vi "Workspace.Initialize.vi"(9 "State Variables in":T1, 10 "Item.Data":T8, 11 "NIVS.Gateway IP Address":string) -> (0 "error out":errorcluster, 3 "State Variables out":T1)   [LabVIEW 2019, in "Protection and Counter Workspace Shared.lvlib"]
uses:
  Protection and Counter Workspace Shared.lvlib
  <vilib>/NI VeriStand/Display Template Support/DisplayTemplateSupport.llb/cluster_Screen Item Settings.ctl
  <vilib>/NI VeriStand/Display Template Support/DisplayTemplateSupport.llb/cluster_Graph Scale Settings.ctl
  <vilib>/NI VeriStand/Display Template Support/DisplayTemplateSupport.llb/cluster_Graph Plot Settings.ctl
  Types/Workspace.State.ctl
  Types/UI.Refs.ctl
  SubModules/CAN-Streaming-Support/Source/Addon/Addon Shared/Types/Type Filter.ctl
  <vilib>/NI VeriStand/Display Template Support/DisplayTemplateSupport.llb/enum_Display Template Handler Minimal To Workspace.ctl
  Types/Workspace.SavedState.ctl
  NationalInstruments.VeriStand.SystemStorage
  <vilib>/NI VeriStand/Execution/Workspace/WorkspaceAPI.ctl
  NationalInstruments.VeriStand.ClientAPI
  <vilib>/NI VeriStand/Display Template Support/DisplayTemplateSupport.llb/enum_Display Template Handler Minimal To Widget Msg.ctl
  <vilib>/NI VeriStand/Execution/Workspace/SystemStateRegEventRef.ctl
  <vilib>/NI VeriStand/Execution/Workspace/Target State Info.ctl
  <vilib>/NI VeriStand/Execution/Workspace/Target State.ctl
  <vilib>/NI VeriStand/Execution/Workspace/SystemStateEventRef.ctl
  SubModules/CAN-Streaming-Support/Source/UIs/Workspace Shared/Types/Host Stream Queue Refs.ctl
  SubModules/CAN-Streaming-Support/Source/UIs/Workspace Shared/Types/Host Stream Queue Type.ctl
  SubModules/CAN-Streaming-Support/Source/UIs/Workspace Shared/Types/Host Stream Queue Command.ctl
  <vilib>/xnet/xnet.llb/XNET Frame CAN.ctl
  <vilib>/xnet/xnet.llb/XNET Frame Type CAN.ctl
  <vilib>/NI VeriStand/Execution/Workspace/NI_VS Workspace ExecutionAPI.lvlib
  SubModules/CAN-Streaming-Support/Source/UIs/Workspace Shared/CAN Stream Support Workspace Shared.lvlib
  SubModules/CAN-Streaming-Support/Source/Addon/Addon Shared/CAN Stream Support Shared.lvlib
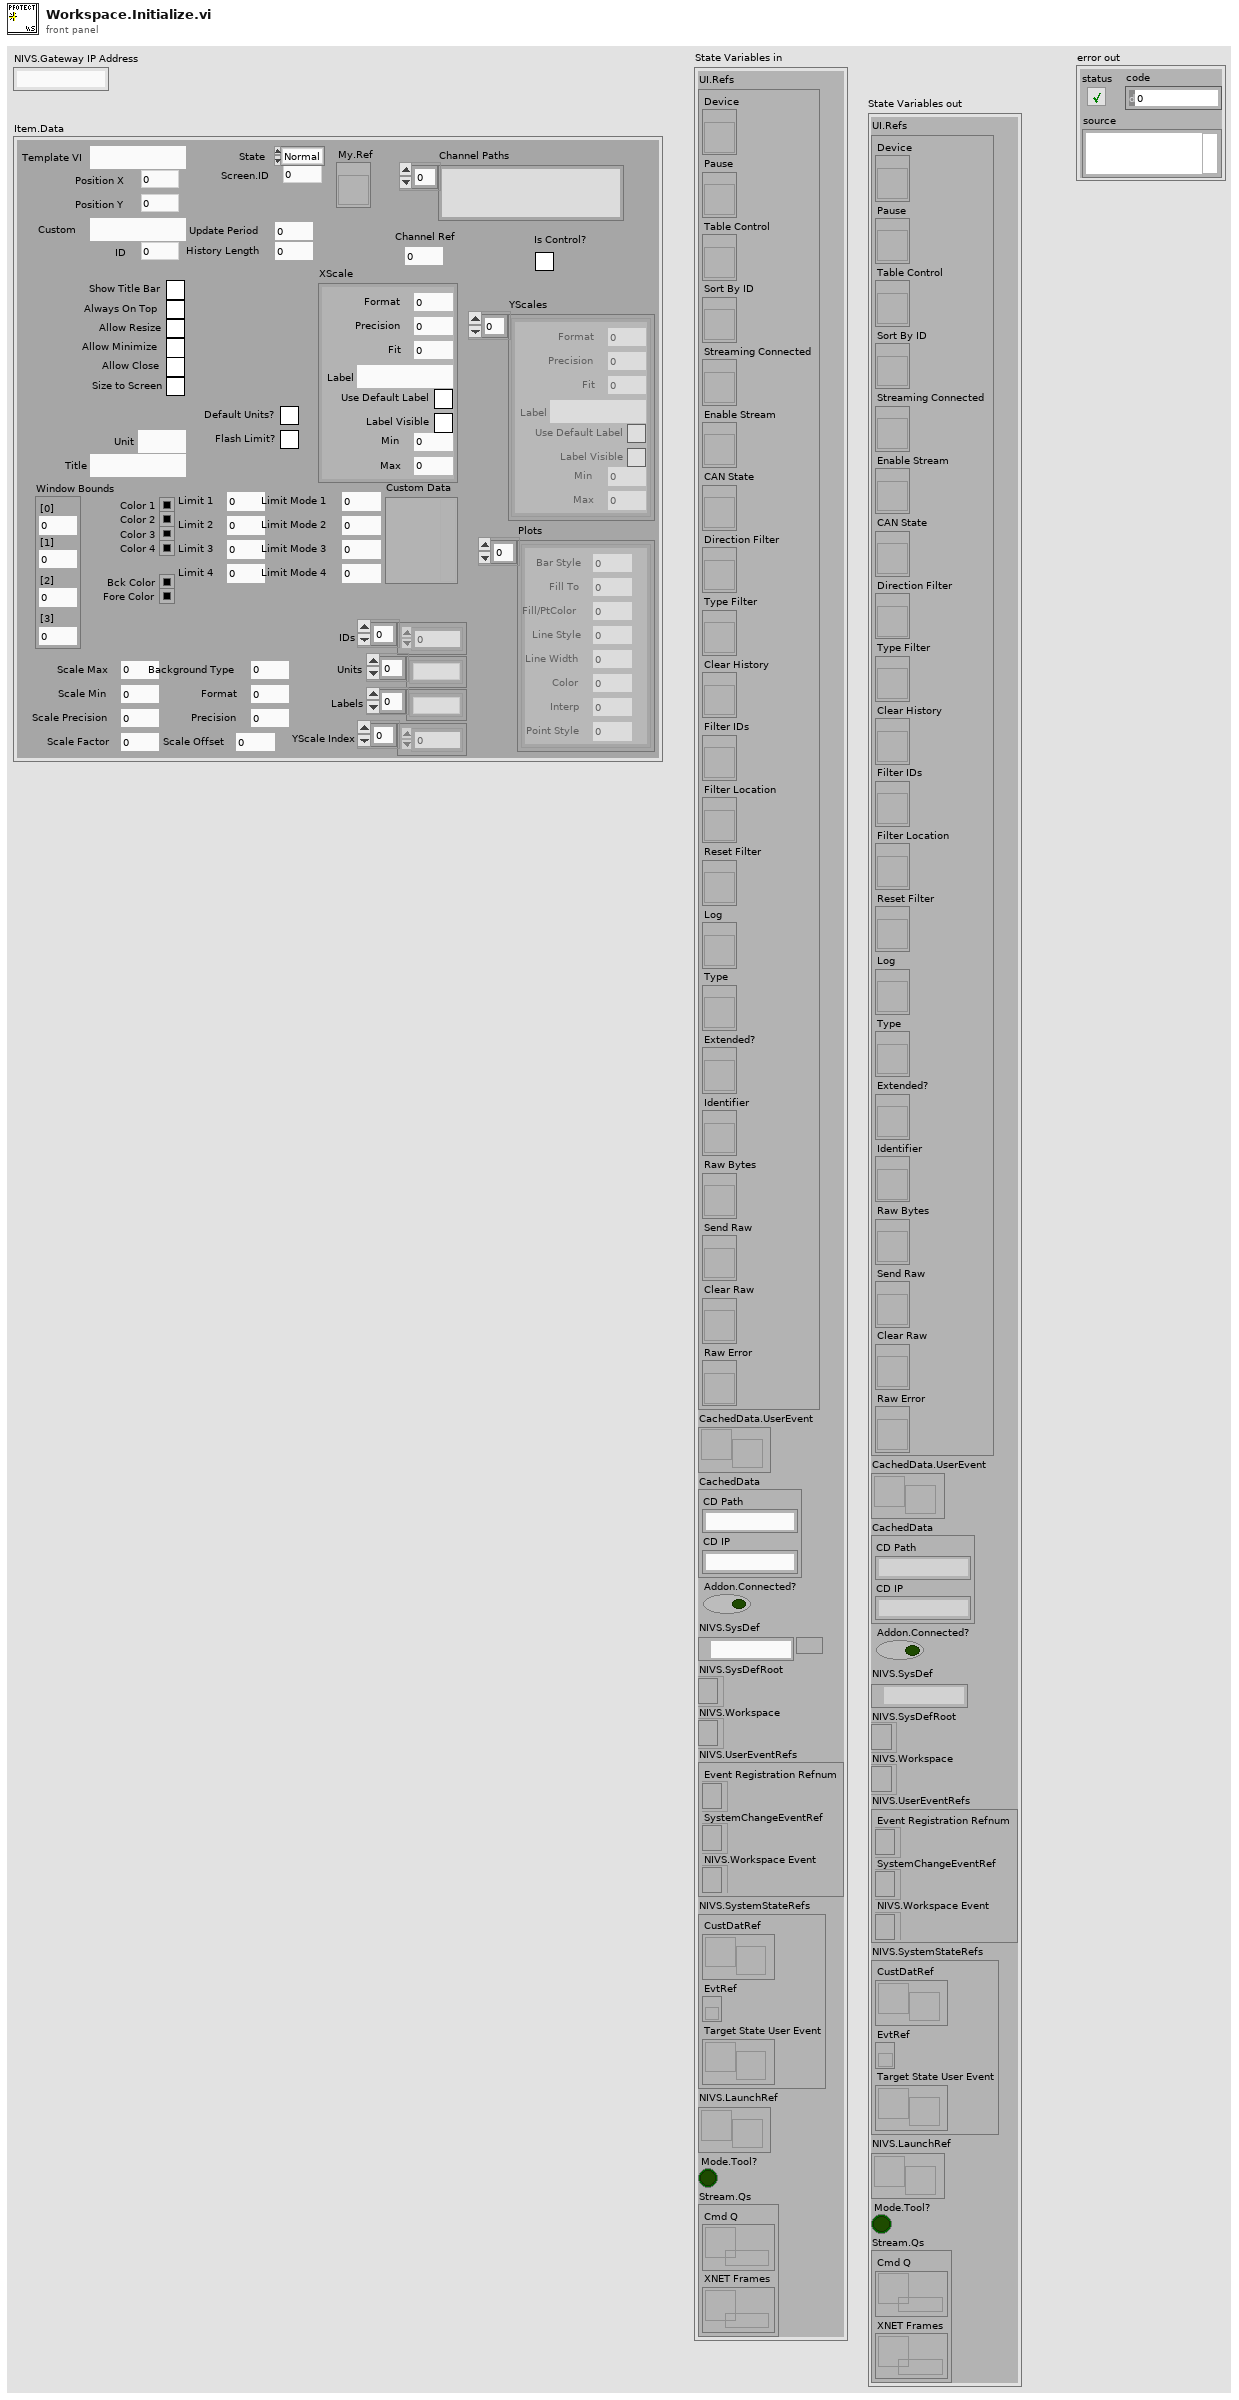
[diagram p1: front panel]
types:
  T1 = typedef "Protection and Counter Workspace Shared.lvlib/Workspace.State.ctl" = cluster{"UI.Refs":T2, "CachedData.UserEvent":refnum<user-event>, "CachedData":T3, "Addon.Connected?":bool, "NIVS.SysDef":path, "NIVS.SysDefRoot":refnum<k24>, "NIVS.Workspace":T4, "NIVS.UserEventRefs":cluster{"Event Registration Refnum":refnum<event-registration>, "SystemChangeEventRef":T5, "NIVS.Workspace Event":refnum<event-registration>}, "NIVS.SystemStateRefs":T6, "NIVS.LaunchRef":refnum<user-event>, "Mode.Tool?":bool, "Stream.Qs":T7}
  T2 = typedef "Protection and Counter Workspace Shared.lvlib/UI.Refs.ctl" = cluster{"Device":refnum<vi>, "Pause":refnum<vi>, "Table Control":refnum<vi>, "Sort By ID":refnum<vi>, "Streaming Connected":refnum<vi>, "Enable Stream":refnum<vi>, "CAN State":refnum<vi>, "Direction Filter":refnum<vi>, "Type Filter":refnum<vi>, "Clear History":refnum<vi>, "Filter IDs":refnum<vi>, "Filter Location":refnum<vi>, "Reset Filter":refnum<vi>, "Log":refnum<vi>, "Type":refnum<vi>, "Extended?":refnum<vi>, "Identifier":refnum<vi>, "Raw Bytes":refnum<vi>, "Send Raw":refnum<vi>, "Clear Raw":refnum<vi>, "Raw Error":refnum<vi>}
  T3 = typedef "Protection and Counter Workspace Shared.lvlib/Workspace.SavedState.ctl" = cluster{"CD Path":string, "CD IP":string}
  T4 = typedef "NI_VS Workspace ExecutionAPI.lvlib/WorkspaceAPI.ctl" = refnum<k24>
  T5 = typedef "NI_VS Workspace ExecutionAPI.lvlib/SystemStateRegEventRef.ctl" = refnum<event-registration>
  T6 = typedef "NI_VS Workspace ExecutionAPI.lvlib/SystemStateEventRef.ctl" = cluster{"CustDatRef":refnum<user-event>, "EvtRef":refnum<k27>, "Target State User Event":refnum<user-event>}
  T7 = typedef "CAN Stream Support Workspace Shared.lvlib/Host Stream Queue Refs.ctl" = cluster{"Cmd Q":refnum<queue>, "XNET Frames":refnum<queue>}
  T8 = typedef "cluster_Screen Item Settings.ctl" = cluster{"Template VI":string, "Position X":i32, "Position Y":i32, "Custom":string, "Show Title Bar":bool, "ID":i32, "Always On Top":bool, "Allow Resize":bool, "Allow Minimize":bool, "Allow Close":bool, "Size to Screen":bool, "Screen.ID":i32, "State":enum16{"Normal", "New"}, "Title":string, "Window Bounds":cluster{"[0]":i16, "[1]":i16, "[2]":i16, "[3]":i16}, "Channel Ref":u64, "Unit":string, "Default Units?":bool, "Flash Limit?":bool, "Color 1":u32, "Color 2":u32, "Color 3":u32, "Color 4":u32, "Bck Color":u32, "Fore Color":u32, "Limit 1":dbl, "Limit 2":dbl, "Limit 3":dbl, "Limit 4":dbl, "Limit Mode 1":i32, "Limit Mode 2":i32, "Limit Mode 3":i32, "Limit Mode 4":i32, "Scale Precision":i32, "Scale Min":dbl, "Scale Max":dbl, "Format":i32, "Precision":i32, "Background Type":i32, "IDs":i32[], "Units":string[], "Labels":string[], "Scale Factor":dbl, "Scale Offset":dbl, "YScale Index":u32[], "XScale":T9, "YScales":T9[], "Plots":T10[], "Update Period":dbl, "History Length":dbl, "My.Ref":refnum<vi>, "Is Control?":bool, "Channel Paths":string[], "Custom Data":variant}
  T9 = typedef "cluster_Graph Scale Settings.ctl" = cluster{"Format":u8, "Precision":u8, "Fit":u8, "Label":string, "Use Default Label":bool, "Label Visible":bool, "Min":dbl, "Max":dbl}
  T10 = typedef "cluster_Graph Plot Settings.ctl" = cluster{"Bar Style":u8, "Fill To":i16, "Fill/PtColor":u32, "Line Style":u8, "Line Width":u8, "Color":u32, "Interp":u8, "Point Style":u8}
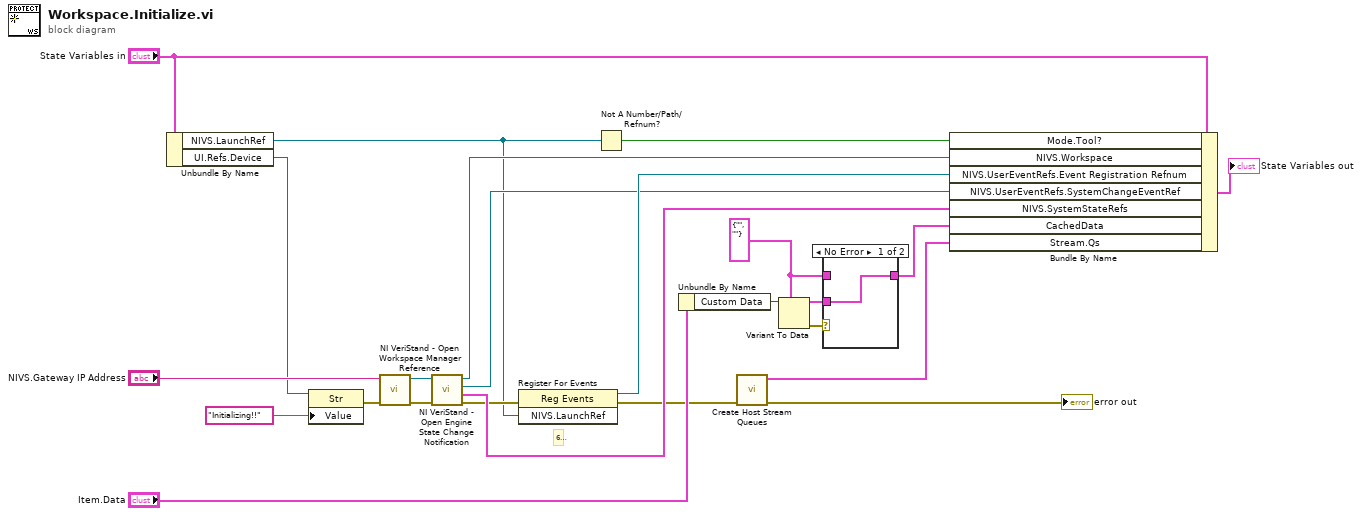
[diagram p0: block diagram]
diagram:
  w12 = T3 {"CD Path"="", "CD IP"=""} ("CachedData")
  # "6."
  n1 = Unbundle By Name("State Variables in") -> ("NIVS.LaunchRef"=w8:refnum<user-event>, "UI.Refs.Device"=w6:refnum<vi>)
  n2 = property class="Str"(reference=w6, "Value"="Initializing!!") -> (error out=w5:errorcluster)  [unwired: 1 in, 1 out]
  n3 = call <vilib>:"NI VeriStand - Open Workspace Manager Reference.vi"("error in (no error)"=w5, "Gateway IP Address (\"\": localhost)"="NIVS.Gateway IP Address") -> ("error out"=w16:errorcluster, "WorkspaceManager"=w21:T4)  [unwired: 8 in]
  n4 = call <vilib>:"NI VeriStand - Open Engine State Change Notification.vi"("error in (no error)"=w16, "WorkspaceManager in"=w21) -> ("error out"=w13:errorcluster, "SystemStateRefs"=w20:T6, "SystemChangeEventRef"=w9:T5, "WorkspaceManager out"=w14:T4)  [unwired: 6 in]
  n5 = register-events(error in=w13, w8) -> (reference out=w10:refnum<event-registration>, error out=w3:errorcluster)  [unwired: 1 in]
  n6 = Not A Number/Path/Refnum?(number/path/refnum=w8) -> (NaN/Path/Refnum?=w7:bool)
  n7 = Unbundle By Name("Item.Data") -> ("Custom Data"=w17:variant)
  n8 = call "Create Host Stream Queues.vi"("error in (no error)"=w3) -> ("error out"=→"error out":errorcluster, "Q Refs"=w1:T7)  [unwired: 9 in]
  n9 = Variant To Data(type=w12, Variant=w17) -> (data=w19:T3, error out=w18:errorcluster)  [unwired: 1 in]
  n10 = case shown="No Error" w18 {
    tunnel: w19 -> [w25 _]
    tunnel: [w25 w26] -> w11
    tunnel: w12 -> [_ w26]
    frame No Error {
    }
    frame Error {
    }
  }
  n11 = Bundle By Name(cluster="State Variables in", "Mode.Tool?"=w7, "NIVS.Workspace"=w14, "NIVS.UserEventRefs.Event Registration Refnum"=w10, "NIVS.UserEventRefs.SystemChangeEventRef"=w9, "NIVS.SystemStateRefs"=w20, "CachedData"=w11, "Stream.Qs"=w1) -> (→"State Variables out":T1)
